vi "TestSCAN_MX5060.vi"(8 "errin":errorcluster) -> (0 "error out":errorcluster, 2 "Tableau 2":refnum<visa-resource-name>[](array[refnum]), 3 "Tableau":string[](array[string]))   [LabVIEW 2020]
doc: "Ce VI te sniff tout les équipement VISA qu'il détect et t'en fait une liste"
uses:
  <vilib>/Instr/_visa.llb/VISA Find Search Mode.ctl
  <vilib>/Instr/_visa.llb/VISA Configure Serial Port (Instr).vi
  <instrlib>/HIOKI BT356X Series/HIOKI BT356X Series.lvlib
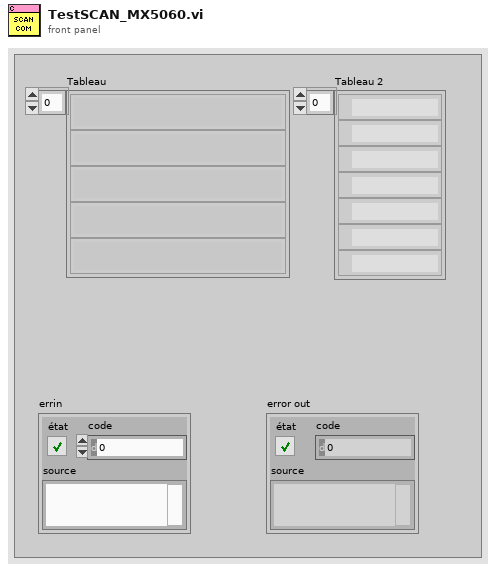
[diagram p1: front panel]
types:
  T1 = typedef "VISA Find Search Mode.ctl" = u32
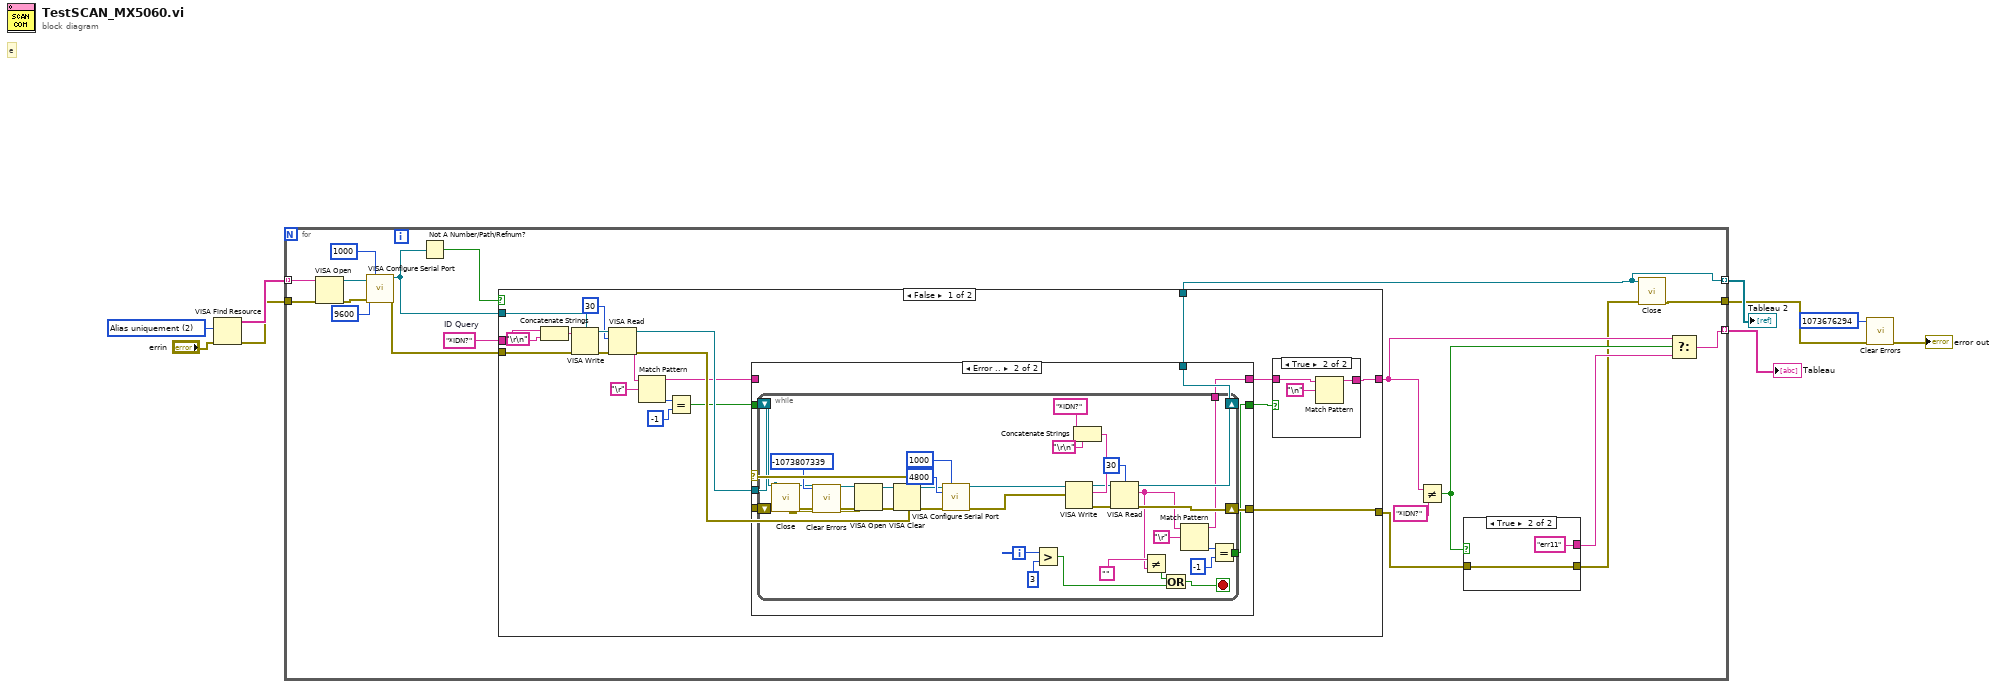
[diagram p0: block diagram]
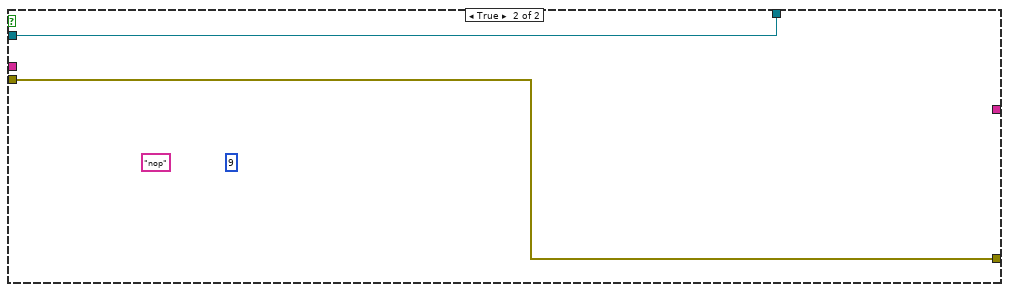
[diagram p4: hidden frame]
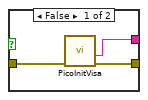
[diagram p5: hidden frame]
diagram:
  w5 = T1 2 items=["Noms canoniques uniquement"=0, "Alias uniquement"=2, "Inclure les alias correspondants"=3, "Inclure tous les alias"=4] ("Search Mode")
  # "e"
  n1 = VISA Find Resource(8:"errin", 10:w5) -> (0:w4:errorcluster, 3:w9:string[])  [unwired: 1 in, 1 out]
  n2 = for {
    tunnel: w9 -> [w28] mode=indexing
    tunnel: [w20] -> w8 mode=indexing
    tunnel: [w13] -> w6 mode=indexing
    tunnel: w4 -> [w27]
    tunnel: [w24] -> w3
    w25 = "*IDN?"  # ID Query
    n3 = VISA Open(error in (no error)=w27, VISA resource name=w28) -> (VISA resource name=w14:refnum<visa-resource-name>, error out=w16:errorcluster)  [unwired: 3 in]
    n4 = call-poly "VISA Configure Serial Port"("VISA resource name"=w14, "timeout (10sec)"=u32 1000, "baud rate (9600)"=u32 9600, "error in (no error)"=w16) -> ("VISA resource name out"=w11:refnum<visa-resource-name>, "error out"=w15:errorcluster)  [unwired: 10 in]
    n5 = Not A Number/Path/Refnum?(number/path/refnum=w11) -> (NaN/Path/Refnum?=w26:bool)
    n6 = case shown="False" w26 {
      tunnel: [w33 w98] -> w18
      tunnel: [w43 _] -> w19
      tunnel: w11 -> [w37 w97]
      tunnel: w25 -> [w42 _]
      tunnel: w15 -> [w40 w98]
      tunnel: [w34 w97] -> w13
      frame False {
        n7 = Concatenate Strings(w42, "\r\n") -> (w46:string)
        n8 = VISA Write(VISA resource name=w37, write buffer=w46, error in (no error)=w40) -> (VISA resource name out=w49:refnum<visa-resource-name>, error out=w48:errorcluster)  [unwired: 1 out]
        n9 = VISA Read(VISA resource name=w49, byte count=u32 30 ("nombre d'octets"), error in (no error)=w48) -> (VISA resource name out=w36:refnum<visa-resource-name>, read buffer=w39:string, error out=w35:errorcluster)  [unwired: 1 out]
        n10 = Match Pattern(string=w39, regular expression="\r") -> (before substring=w30:string, offset past match=w38:i32)  [unwired: 1 in, 2 out]
        n11 = Equal?(x=w38, y=-1) -> (x = y?=w31:bool)
        n12 = case shown="Error .." w35 {
          tunnel: w36 -> [w53 w54]
          tunnel: w35 -> [w52 w55]
          tunnel: [w53 w59] -> w34
          tunnel: [w52 w58] -> w33
          tunnel: [w51 w57] -> w32
          tunnel: w31 -> [w51 _]
          tunnel: w30 -> [w50 _]
          tunnel: [w50 w56] -> w29
          frame No Error {
          }
          frame Error {
            n13 = while {
              tunnel: [w82] -> w57
              tunnel: [w81] -> w56
              shift-right: [w86] -> w58
              shift-left: w55 -> [w77]
              shift-right: [w87] -> w59
              shift-left: w54 -> [w76]
              i -> [w66]
              stop <- w63 stop-if-true
              n14 = call <instrlib>:"Close.vi"("error in (no error)"=w77, "VISA resource name"=w76) -> ("error out"=w75:errorcluster)  [unwired: 9 in]
              n15 = call <vilib>:"Clear Errors.vi"("error in (no error)"=w75, "specific error code to clear (0: all)"=-1073807339) -> ("error out"=w79:errorcluster)  [unwired: 4 in, 1 out]
              n16 = VISA Open(error in (no error)=w79, VISA resource name=w76) -> (VISA resource name=w74:refnum<visa-resource-name>, error out=w73:errorcluster)  [unwired: 3 in]
              n17 = VISA Clear(VISA resource name=w74, error in (no error)=w73) -> (VISA resource name out=w71:refnum<visa-resource-name>, error out=w72:errorcluster)
              n18 = call-poly "VISA Configure Serial Port"("VISA resource name"=w71, "timeout (10sec)"=u32 1000, "baud rate (9600)"=u32 4800, "error in (no error)"=w72) -> ("VISA resource name out"=w62:refnum<visa-resource-name>, "error out"=w61:errorcluster)  [unwired: 10 in]
              n19 = Greater?(x=w66, y=3) -> (0:w64:bool)
              n20 = Concatenate Strings("*IDN?" ("chaîne"), "\r\n") -> (w90:string)
              n21 = VISA Write(VISA resource name=w62, write buffer=w90, error in (no error)=w61) -> (VISA resource name out=w70:refnum<visa-resource-name>, error out=w92:errorcluster)  [unwired: 1 out]
              n22 = VISA Read(VISA resource name=w70, byte count=u32 30 ("nombre d'octets"), error in (no error)=w92) -> (VISA resource name out=w87:refnum<visa-resource-name>, read buffer=w68:string, error out=w86:errorcluster)  [unwired: 1 out]
              n23 = Not Equal?(x="", y=w68) -> (x != y?=w67:bool)
              n24 = Or(x=w67, y=w64) -> (x .or. y?=w63:bool)
              n25 = Match Pattern(string=w68, regular expression="\r") -> (before substring=w81:string, offset past match=w83:i32)  [unwired: 1 in, 2 out]
              n26 = Equal?(x=w83, y=-1) -> (x = y?=w82:bool)
            }
          }
        }
        n27 = case shown="True" w32 {
          tunnel: [w93 w95] -> w43
          tunnel: w29 -> [w93 w94]
          frame False {
          }
          frame True {
            n28 = Match Pattern(string=w94, regular expression="\n") -> (before substring=w95:string)  [unwired: 1 in, 3 out]
          }
        }
      }
      frame True {
        (unwired) 9 ("offset past match")
        (unwired) "nop" ("read buffer")
      }
    }
    n29 = Not Equal?(x=w19, y="*IDN?") -> (x != y?=w22:bool)
    n30 = case shown="True" w22 {
      tunnel: [w101 w102] -> w17
      tunnel: [w100 "err11" ("data out")] -> w21
      tunnel: w18 -> [w99 w102]
      frame False {
        n31 = call <userlib>:"PicoInitVisa.vi"("errin"=w99) -> ("sortie d'erreur"=w101:errorcluster, "buffer de lecture 2"=w100:string)  [unwired: 7 in, 2 out]
      }
      frame True {
      }
    }
    n32 = call <instrlib>:"Close.vi"("error in (no error)"=w17, "VISA resource name"=w13) -> ("error out"=w24:errorcluster)  [unwired: 9 in]
    n33 = Select(t=w19, s=w22, f=w21) -> (s? t:f=w20:string)
  }
  "Tableau" <- w8
  "Tableau 2" <- w6
  n34 = call <vilib>:"Clear Errors.vi"("error in (no error)"=w3, "specific error code to clear (0: all)"=1073676294) -> ("error out"=→"error out":errorcluster)  [unwired: 4 in, 1 out]
